vi "Day 6 Task 1.vi"() -> ()   [LabVIEW 2018]
panel:
  out "time string":string
  out "Numeric":i32
  out "No. fish":i32
  out "After N days":u8[](array[numeric])
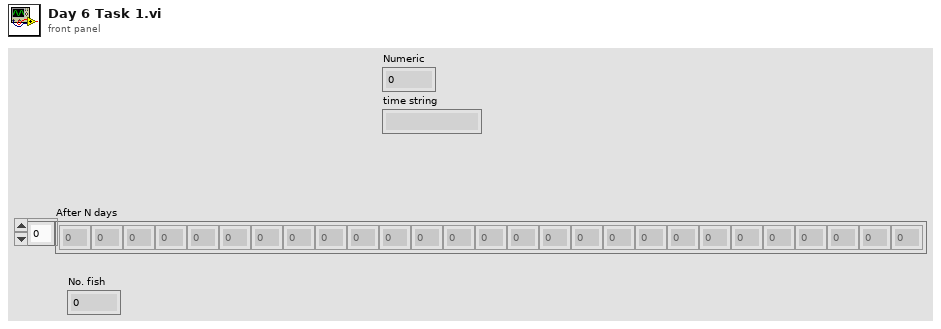
[diagram p1: front panel]
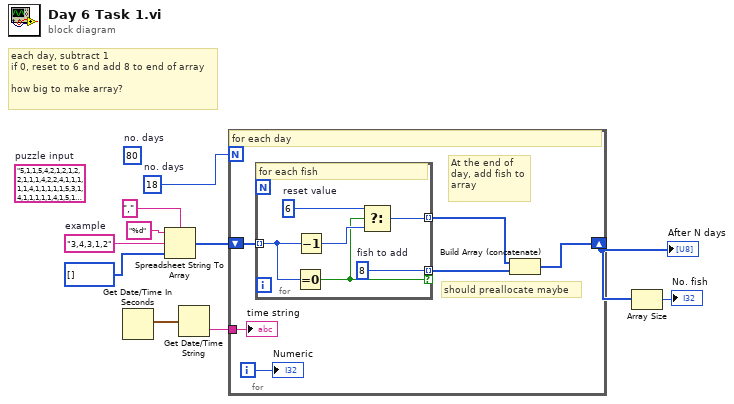
[diagram p0: block diagram]
diagram:
  (unwired) 80  # no. days
  (unwired) "5,1,1,5,4,2,1,2,1,2,2,1,1,1,4,2,2,4,1,1,1,1,1,4,1,1,1,1,1,5,3,1,4,1,1,1,1,1,4,1,5,1,1,1,4,1,2,2,3,1,5,1,1,5,1,1,5,4,1,1,1,4,3,1,1,1,3,1,5,5,1,1,1,1,5,3,2,1,2,3,1,5,1,1,4,1,1,2,1,5,1,1,1,1,5,4,5,1,3,1,3,3,5,5,1,3,1,5,3,1,1,4,2,3,3,1,2,4,1,1,1,1,1,1,1,2,1,1,4,1,3,2,5,2,1,1,1,4,2,1,1,1,4,2,4,1,1,1,1,4,1,3,5,5,1,2,1,3,1,1,4,1,1,1,1,2,1,1,4,2,3,1,1,1,1,1,1,1,4,5,1,1,3,1,1,2,1,1,1,5,1,1,1,1,1,3,2,1,2,4,5,1,5,4,1,1,3,1,1,5,5,1,3,1,1,1,1,4,4,2,1,2,1,1,5,1,1,4,5,1,1,1,1,1,1,1,1,1,1,3,1,1,1,1,1,4,2,1,1,1,2,5,1,4,1,1,1,4,1,1,5,4,4,3,1,1,4,5,1,1,3,5,3,1,2,5,3,4,1,3,5,4,1,3,1,5,1,4,1,1,4,2,1,1,1,3,2,1,1,4"  # puzzle input
  w1 = 18  # no. days
  w2 = "3,4,3,1,2"  # example
  # "each day, subtract 1\nif 0, reset to 6 and add 8 to end of array\n\nhow big to make array?"
  n1 = Get Date/Time In Seconds() -> (seconds since 1Jan1904=w4:timestamp)
  n2 = Spreadsheet String To Array(delimiter (Tab)=",", format string="%d", spreadsheet string=w2, array type (2D Dbl)=u8[] []) -> (array=w7:u8[])
  n3 = Get Date/Time String(seconds (now)=w4) -> (time string=w3:string)  [unwired: 2 in, 1 out]
  n4 = for {
    N: w1 -> [_]
    shift-right: [w13] -> w6
    shift-left: w7 -> [w16]
    tunnel: w3 -> [w11]
    i -> [w12]
    # "should preallocate maybe"
    # "At the end of day, add fish to array"
    # "for each day"
    n5 = for {
      tunnel: w16 -> [w21] mode=indexing
      tunnel: [w22] -> w14 mode=indexing if=w18
      tunnel: [w17] -> w15 mode=indexing
      w20 = u8 6  # reset value
      w22 = u8 8  # fish to add
      # "for each fish"
      n6 = Equal To 0?(x=w21) -> (x = 0?=w18:bool)
      n7 = Decrement(x=w21) -> (x-1=w19:u8)
      n8 = Select(t=w20, s=w18, f=w19) -> (s? t:f=w17:u8)
    }
    n9 = Build Array (concatenate)(w15, w14) -> (w13:u8[])
    "Numeric" <- w12
    "time string" <- w11
  }
  "After N days" <- w6
  n10 = Array Size(array=w6) -> (size(s)=→"No. fish":i32)
